vi "kinect.vi"() -> ()   [LabVIEW 2013]
uses:
  <vilib>/University of Leeds/Kinesthesia Toolkit for Microsoft Kinect/_Polymorphic Configure/Event-Skeleton and Video.vi
  <vilib>/University of Leeds/Kinesthesia Toolkit for Microsoft Kinect/_Polymorphic Close/Close-Skeleton and Video.vi
  <vilib>/University of Leeds/Kinesthesia Toolkit for Microsoft Kinect/_Polymorphic Read/Read-Skeleton and Video.vi
panel:
  out "Esqueleto 3D":refnum<vi>(3d-picture)
  in  "?":bool
  out "X Y Z  Distancia entre punto 1 y 2":dbl[](array[numeric])
  out "Angulo entre punto 1 y 2":dbl
  in  "Punto 2":T1(ring)
  in  "Punto 1":T1(ring)
  out "Camara":picture
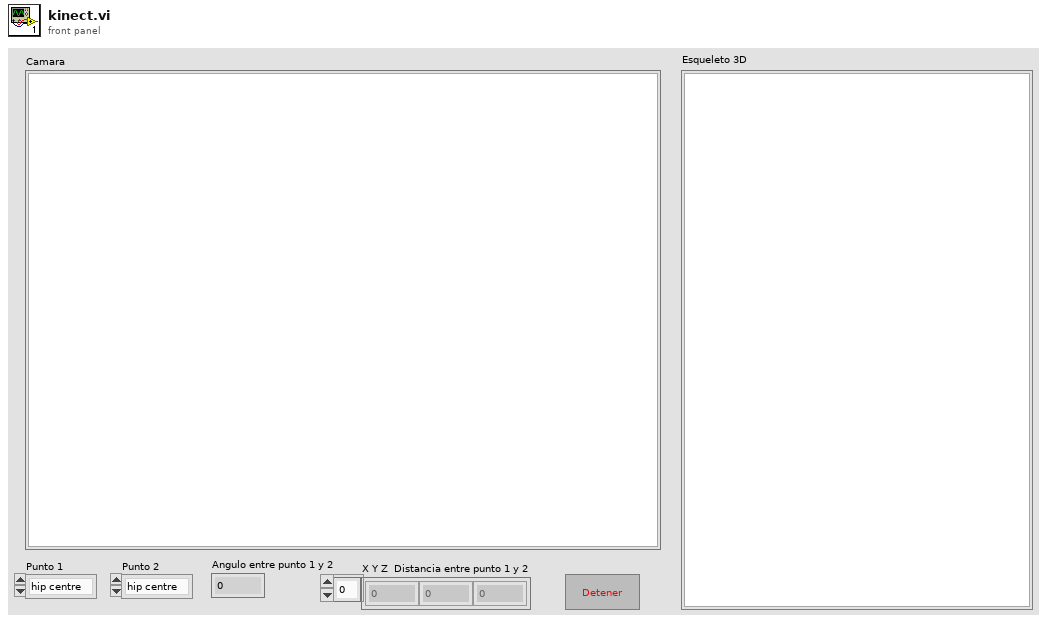
[diagram p1: front panel]
types:
  T1 = enum16{"hip centre", "spine", "shoulder centre", "head", "shoulder left", "elbow left", "wrist left", "hand left", "shoulder right", "elbow right", "wrist right", "hand right", "hip left", "knee left", "ankle left", "foot left", "hip right", "knee right", "ankle right", "foot right"}
  T2 = cluster{cluster{"reference out":refnum<k24>, "KinectSensors":refnum<k24>}, "get_Item":refnum<k24>}
  T3 = cluster{"reference out":refnum<k24>, "KinectSensors":refnum<k24>, "SkeletonStream":refnum<k24>, "ColorStream":refnum<k24>, refnum<k24>[], "get_Item":refnum<k24>}
  T4 = cluster{"Scene":refnum<vi>, "Joints":refnum<vi>[], "Bones":refnum<vi>[]}
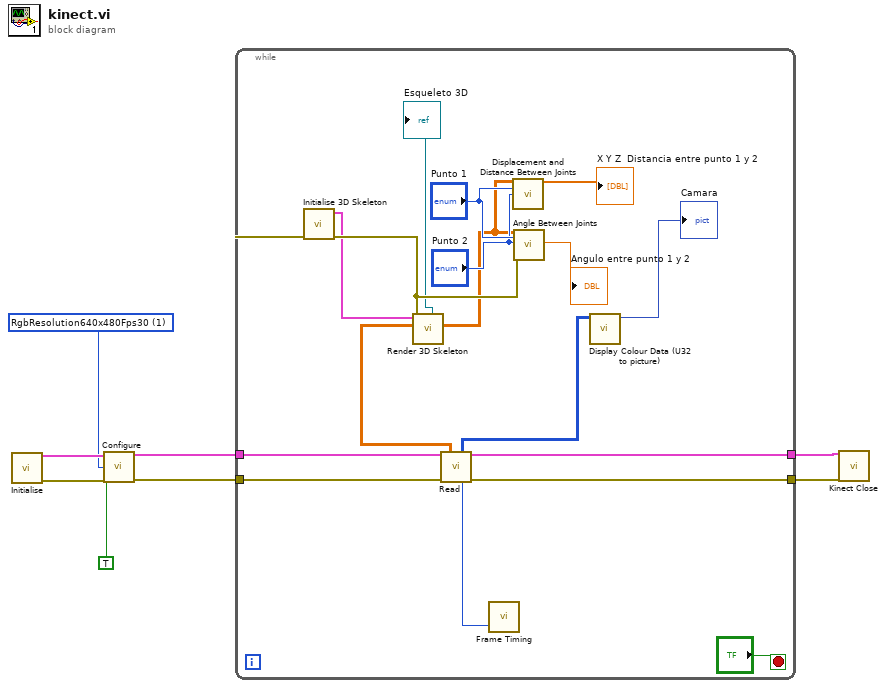
[diagram p0: block diagram]
diagram:
  w2 = 1 items=["Undefined", "RgbResolution640x480Fps30", "RgbResolution1280x960Fps12", "YuvResolution640x480Fps15", "RawYuvResolution640x480Fps15"] ("RGB Stream Format")
  n1 = call <vilib>:"Initialise.vi"() -> ("Kinect References out"=w8:T2, "error out"=w7:errorcluster)  [unwired: 14 in]
  n2 = call-poly <vilib>:"Configure.vi"("Kinect References in"=w8, "RGB Stream Format"=w2, "Skeleton Smoothing"=TRUE, "error in"=w7) -> ("Kinect References out"=w6:T3, "error out"=w5:errorcluster)  [unwired: 10 in]
  n3 = while {
    tunnel: w6 -> [w25]
    tunnel: w5 -> [w24]
    tunnel: [w20] -> w4
    tunnel: [w19] -> w3
    stop <- "?" stop-if-true
    n4 = call <vilib>:"Initialise 3D Skeleton.vi"("error in (no error)"=w24) -> ("error out"=w16:errorcluster, "Scene & Skeleton Refs"=w9:T4)  [unwired: 9 in]
    n5 = call-poly <vilib>:"Read.vi"("Kinect References in"=w25, "error in (no error)"=w24) -> ("Primary Skeleton Array"=w23:dbl[][], "Colour output array (U24, RGB)"=w22:u32[][], "Kinect References out"=w20:T3, "Timestamp"=w18:u32, "error out"=w19:errorcluster)  [unwired: 9 in]
    n6 = call <vilib>:"Render 3D Skeleton.vi"("error in (no error)"=w16, "Array of Joint Positions"=w23, "Scene & Skeleton Refs In"=w9) -> ("Array of Joint Positions Out"=w13:dbl[][], "Scene Out"=→"Esqueleto 3D":refnum<vi>)  [unwired: 5 in, 2 out]
    n7 = call <vilib>:"Frame Timing.vi"("Skeleton Frame\nTimestamp"=w18) -> ()  [unwired: 1 in, 5 out]
    n8 = call <vilib>:"Displacement and Distance Between Joints.vi"("Array of Joint Positions"=w13, "Joint 1"="Punto 1", "Joint 2"="Punto 2") -> ("X Y Z Displacement Between Joints 1 and 2"=→"X Y Z  Distancia entre punto 1 y 2":dbl[])  [unwired: 11 in, 1 out]
    n9 = call <vilib>:"Angle Between Joints.vi"("Array of Joint Positions"=w13, "Joint 1"="Punto 1", "Joint 2"="Punto 2", "error in (no error)"=w16) -> ("Angle Between Joints (degrees)"=→"Angulo entre punto 1 y 2":dbl)  [unwired: 10 in, 5 out]
    n10 = call <vilib>:"Display Colour Data (U32 to picture).vi"("Colour output array (U24, RGB)"=w22) -> ("new picture"=→"Camara":picture)  [unwired: 10 in]
  }
  n11 = call-poly <vilib>:"Kinect Close.vi"("Kinect References in"=w4, "error in"=w3) -> ()  [unwired: 13 in, 1 out]
